vi "Set_VBAT.vi"() -> ()   [LabVIEW 2015]
panel:
  out "Delay (s)":dbl
  out "Voltage":dbl
  in  "error in (no error)":errorcluster
  in  "delay (s)":string="0"
  in  "Voltage":string="0"
  out "error out":errorcluster
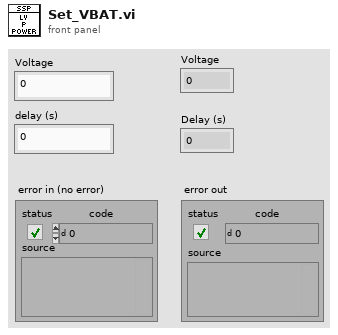
[diagram p1: front panel]
types:
  T1 = enum32{"invalid app kind", "Development System", "Run Time System", "Student Edition", "Embedded LabVIEW", "Evaluation", "Custom"}
  T2 = enum32{"Invalid", "Standard", "Closed", "Hidden", "Minimized", "Maximized"}
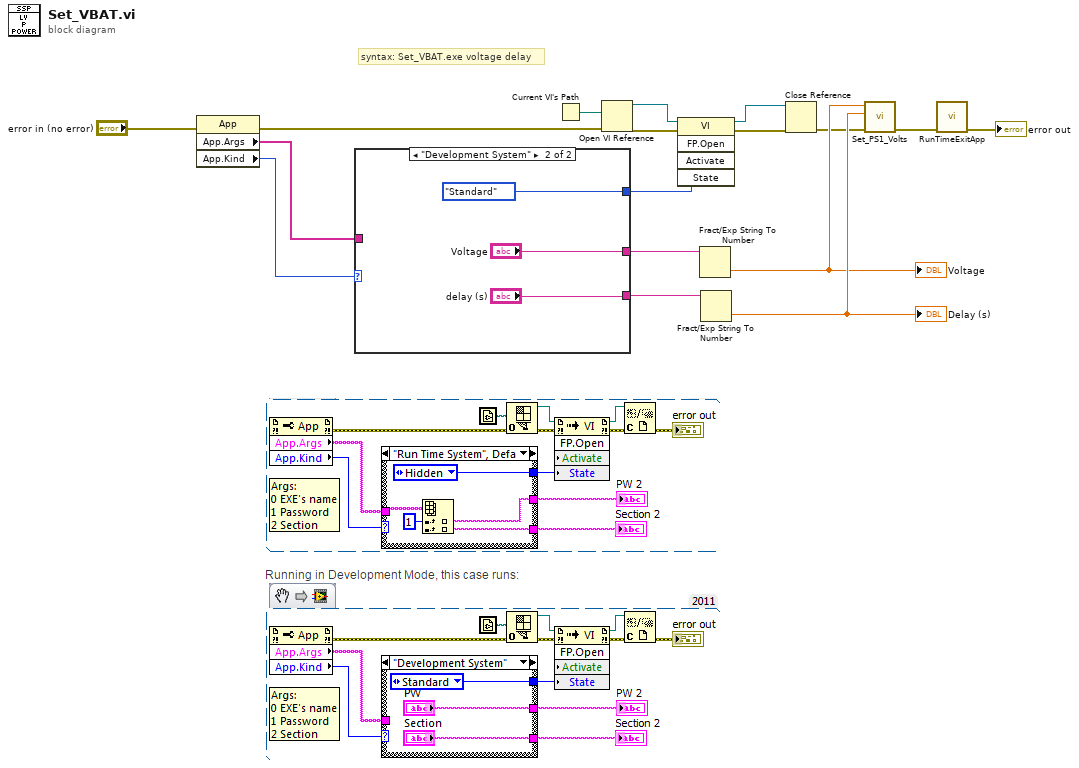
[diagram p0: block diagram]
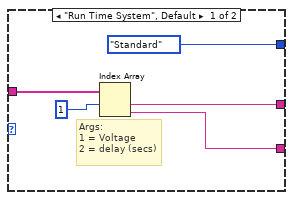
[diagram p2: hidden frame]
diagram:
  # "syntax: Set_VBAT.exe voltage delay"
  n1 = property class="App"(error in="error in (no error)") -> (error out=w12:errorcluster, "App.Args"=w14:string[], "App.Kind"=w15:T1)  [unwired: 1 in, 1 out]
  n2 = case shown="\"Development System\"" w15 {
    tunnel: w14 -> [w18 _]
    tunnel: [w20 "Voltage"] -> w11
    tunnel: [w19 "delay (s)"] -> w10
    tunnel: [T2."Standard" ("State") T2."Standard" ("State")] -> w6
    frame "Run Time System", Default {
      # "Args:\n1 = Voltage\n2 = delay (secs)"
      n3 = Index Array(array=w18, index #1=1 ("index")) -> (element #1=w20:string, element #2=w19:string)  [unwired: 1 in]
    }
    frame "Development System" {
    }
  }
  n4 = Current VI's Path() -> (path=w13:path)
  n5 = Open VI Reference(vi path=w13, error in (no error)=w12) -> (vi reference=w9:refnum<vi>, error out=w7:errorcluster)  [unwired: 4 in]
  n6 = invoke class="VI" method="FP.Open"(reference=w9, error in=w7, "State"=w6) -> (reference out=w5:refnum<vi>, error out=w8:errorcluster)  [unwired: 2 in, 3 out]
  n7 = Fract/Exp String To Number(string=w11) -> (number=w16:dbl)  [unwired: 3 in, 1 out]
  "Voltage" <- w16
  n8 = Fract/Exp String To Number(string=w10) -> (number=w17:dbl)  [unwired: 3 in, 1 out]
  "Delay (s)" <- w17
  n9 = Close Reference(reference=w5, error in (no error)=w8) -> (error out=w1:errorcluster)
  n10 = call "Set_PS1_Volts.vi"("Output Voltage"=w16, "delay (secs)"=w17, "error in"=w1) -> ("error out"=w2:errorcluster)  [unwired: 5 in, 2 out]
  n11 = call "RunTimeExitApp.vi"("error in (no error)"=w2) -> ("error out"=→"error out":errorcluster)  [unwired: 10 in]
